vi "daq_start.vi"(8 "error in":errorcluster, 11 "Tasks":T1) -> (0 "error out":errorcluster)   [LabVIEW 2010]
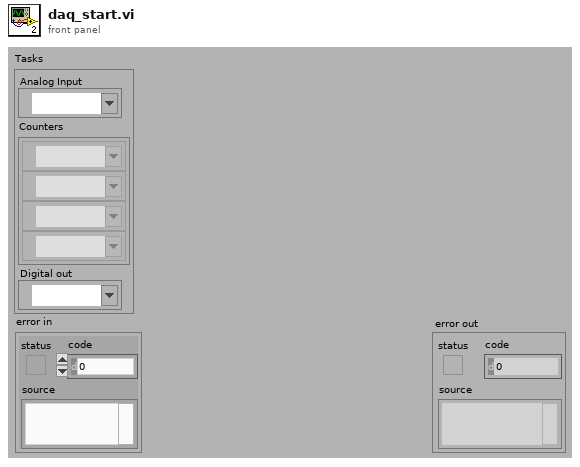
[diagram p1: front panel]
types:
  T1 = cluster{"Analog Input":refnum<k21>, "Counters":refnum<k21>[], "Digital out":refnum<k21>}
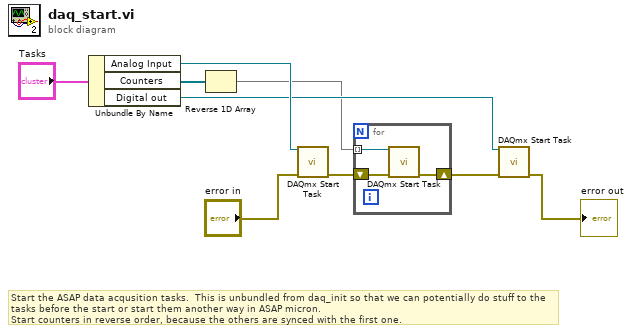
[diagram p0: block diagram]
diagram:
  # "Start the ASAP data acqusition tasks.  This is unbundled from daq_init so that we can potentially do stuff to the tasks before the start or start them another way in ASAP micron.\nStart counters in reverse order, because the others are synced with the first one."
  n1 = Unbundle By Name("Tasks") -> ("Analog Input"=w8:refnum<k21>, "Counters"=w2:refnum<k21>[], "Digital out"=w4:refnum<k21>)
  n2 = Reverse 1D Array(array=w2) -> (reversed array=w1:refnum<k21>[])
  n3 = call <vilib>:"DAQmx Start Task.vi"("task/channels in"=w8, "error in"="error in") -> ("error out"=w6:errorcluster)  [unwired: 13 out]
  n4 = for {
    shift-right: [w11] -> w3
    shift-left: w6 -> [w12]
    tunnel: w1 -> [w10] mode=indexing
    n5 = call <vilib>:"DAQmx Start Task.vi"("task/channels in"=w10, "error in"=w12) -> ("error out"=w11:errorcluster)  [unwired: 13 out]
  }
  n6 = call <vilib>:"DAQmx Start Task.vi"("task/channels in"=w4, "error in"=w3) -> ("error out"=→"error out":errorcluster)  [unwired: 13 out]
